vi "enable_channel_ASIC.vi"(4 "Clip_sel_b":u32, 5 "maj/sum":bool, 6 "Ib_clipVb":u32, 7 "Att gain":u32=4095, 8 "error in":errorcluster, 9 "Channel":u32, 10 "id_in":i32, 11 "connection ID":refnum<k5>) -> (0 "error out":errorcluster, 1 "id_out":i32, 3 "connection ID out":refnum<k5>)   [LabVIEW 2012]
doc: "This VI sends a command to the Integration Board and provides the received data when necessary."
panel:
  out "data out serial":string
  out "data read value":u32=72
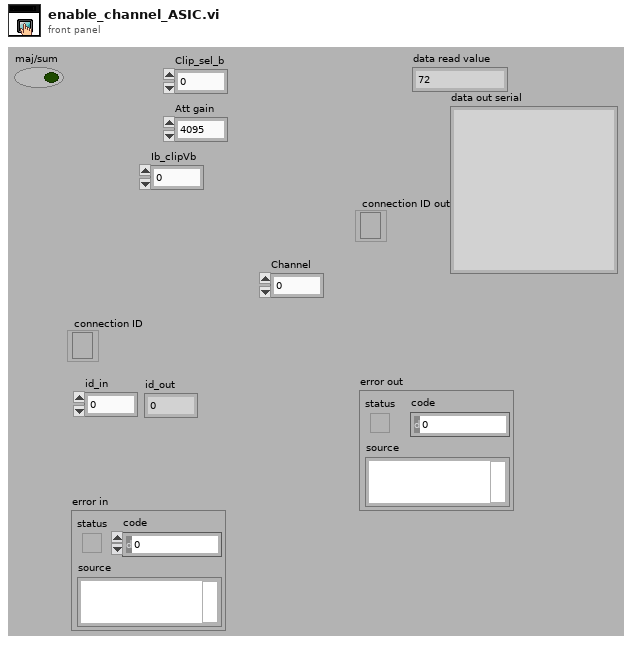
[diagram p1: front panel]
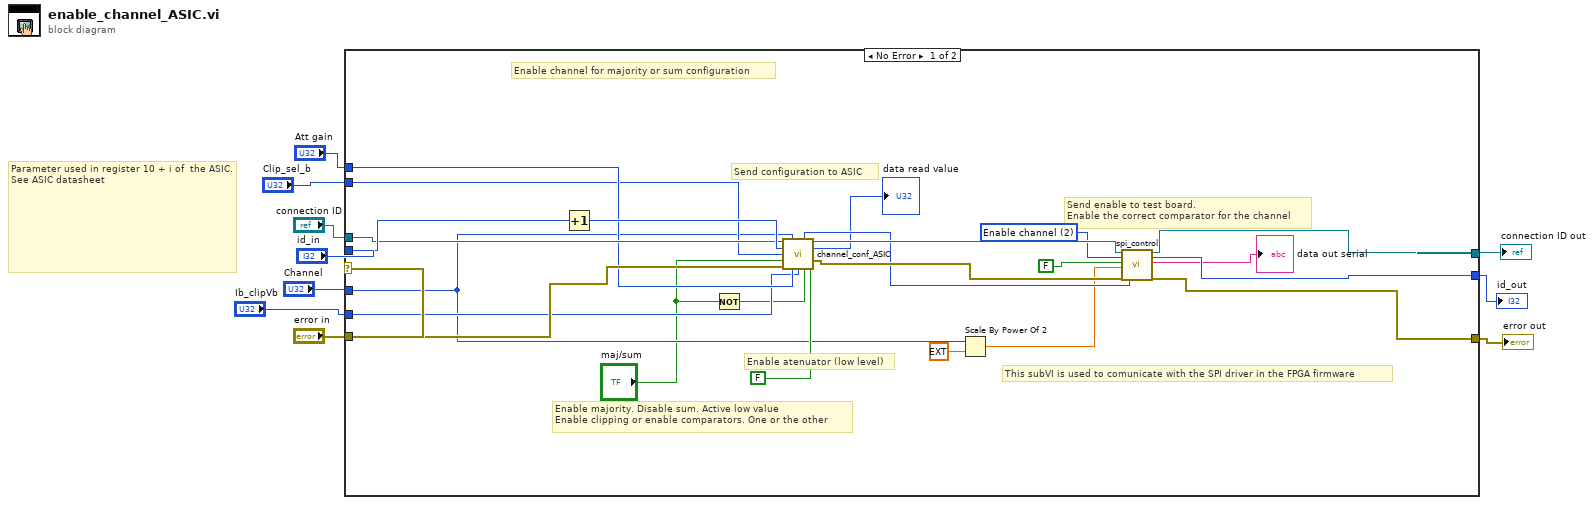
[diagram p0: block diagram]
diagram:
  # "Parameter used in register 10 + i of  the ASIC. See ASIC datasheet"
  n1 = case shown="No Error" "error in" {
    tunnel: "id_in" -> [w26 w34]
    tunnel: "error in" -> [w24 w35]
    tunnel: "connection ID" -> [w25 w36]
    tunnel: [w22 w35] -> w8
    tunnel: [w23 w36] -> w7
    tunnel: "Channel" -> [w15 _]
    tunnel: [w21 w34] -> w5
    tunnel: "Att gain" -> [w19 _]
    tunnel: "Ib_clipVb" -> [w18 _]
    tunnel: "Clip_sel_b" -> [w17 _]
    frame No Error {
      w29 = u16 2 items=["Attenuation", "Clipping", "Enable channel", "Delay line", "ASIC"] ("Device")
      # "This subVI is used to comunicate with the SPI driver in the FPGA firmware"
      # "Send enable to test board. \nEnable the correct comparator for the channel"
      # "Enable majority. Disable sum. Active low value\nEnable clipping or enable comparators. One or the other"
      # "Enable atenuator (low level)"
      # "Send configuration to ASIC"
      # "Enable channel for majority or sum configuration"
      n2 = Increment(x=w26) -> (x+1=w33:i32)
      n3 = Not(x="maj/sum") -> (.not. x?=w11:bool)
      n4 = call "channel_conf_ASIC.vi"("connection ID"=w25, "Ring"=w15, "Id in"=w33, "Clip_sel_b"=w17, "CompBuf_en_b"="maj/sum", "error out"=w24, "Att gain"=w19, "Ib_ClipVb"=w18, "Clip_en_b"=w11, "Att_en_b"=FALSE) -> ("Id out"=w30:i32, "connection ID out"=w32:refnum<k5>, "data read value"=→"data read value":u32, "error out 2"=w31:errorcluster)  [unwired: 1 in, 1 out]
      n5 = Scale By Power Of 2(n=w15, x=ext 1.0) -> (x*2^n=w16:ext)
      n6 = call "spi_control.vi"("connection ID"=w32, "Device"=w29, "Read/#write"=FALSE, "Data"=w16, "error out 3"=w31, "Id in"=w30) -> ("connection ID out"=w23:refnum<k5>, "Id out"=w21:i32, "data out serial"=→"data out serial":string, "error out 2"=w22:errorcluster)  [unwired: 6 in, 4 out]
    }
    frame Error {
    }
  }
  "error out" <- w8
  "connection ID out" <- w7
  "id_out" <- w5
